vi "Acq-module.vi"(7 "IntermediateFIFO":refnum<k21>="FIFO0", 8 "NumChannels":T1, 9 "SamplingRate0":u16=10000, 11 "Cluster in":T3) -> (3 "cluster out":T4)   [LabVIEW 2013]
uses:
  ctl.ctl
  N Channels.ctl
  <vilib>/rvi/DataTransferAndStorage/Container/Common/niFpgaContainerExecOnDevCompGetState.vi
  <vilib>/rvi/FIFO/Fifo_Resource/nirvififoEmulationWriteFpgaImpl.vi
  <vilib>/rvi/DataTransferAndStorage/Container/Common/niFpgaContainerGetUniqueNameForEmu.vi
  <vilib>/rvi/interface/RandomDataEmulation/nirviRandomDataFPGAFIFO.vi
  <vilib>/rvi/interface/RandomDataEmulation/niFpgaRandomDataHandleErrors.vi
  <vilib>/rvi/eio/common/nirviEmuReportErrorAndStop.vi
  <vilib>/rvi/Emulation/niFpgaSctlEmulationGetInTimedLoop.vi
  <vilib>/rvi/Emulation/niFpgaProcessEmulError.vi
  GlobalReg.vi
  <vilib>/rvi/eio/common/nirviEmuTemplateMethod_errors.vi
  <vilib>/rvi/DataTransferAndStorage/Container/XNode/niFpgaContainer.xnode
  <vilib>/rvi/FIFO/Fifo_Resource/niFpgaFifoEmulationRefIn.vi
  <vilib>/eio/EIONode/EIONode.xnode
panel:
  out "Analog Out Cluster":T2
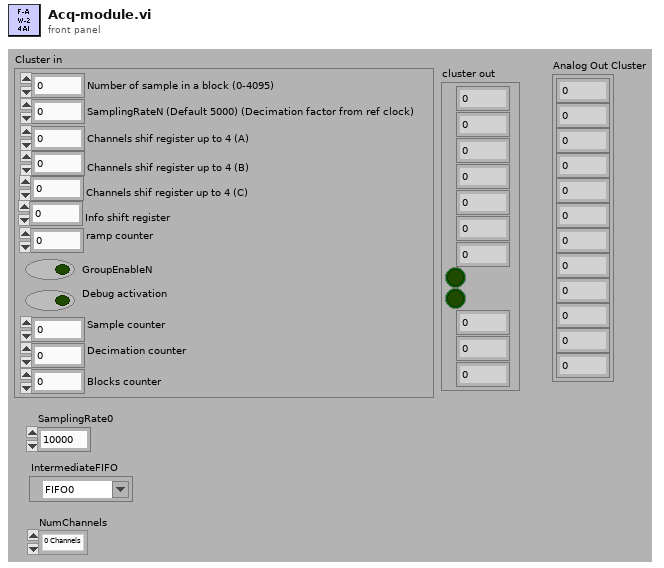
[diagram p1: front panel]
types:
  T1 = typedef "N Channels.ctl" = enum16{"0 Channels", "1 Channels", "2 Channels", "3 Channels", "4 Channels", "5 Channels", "6 Channels", "7 Channels", "8 Channels", "9 Channels", "10 Channels", "11 Channels", "12 Channels"}
  T2 = cluster{i16, i16, i16, i16, i16, i16, i16, i16, i16, i16, i16, i16}
  T3 = typedef "ctl.ctl" = cluster{"Number of sample in a block (0-4095)":u16, "SamplingRateN (Default 5000) (Decimation factor from ref clock)":u16, "Channels shif register up to 4 (A) ":u64, "Channels shif register up to 4 (B) ":u64, "Channels shif register up to 4 (C) ":u64, "Info shift register":u64, "ramp counter":i16, "GroupEnableN":bool, "Debug activation":bool, "Sample counter ":u64, "Decimation counter":u16, "Blocks counter":u16}
  T4 = cluster{u16, u16, u64, u64, u64, u64, i16, bool, bool, u64, u16, u16}
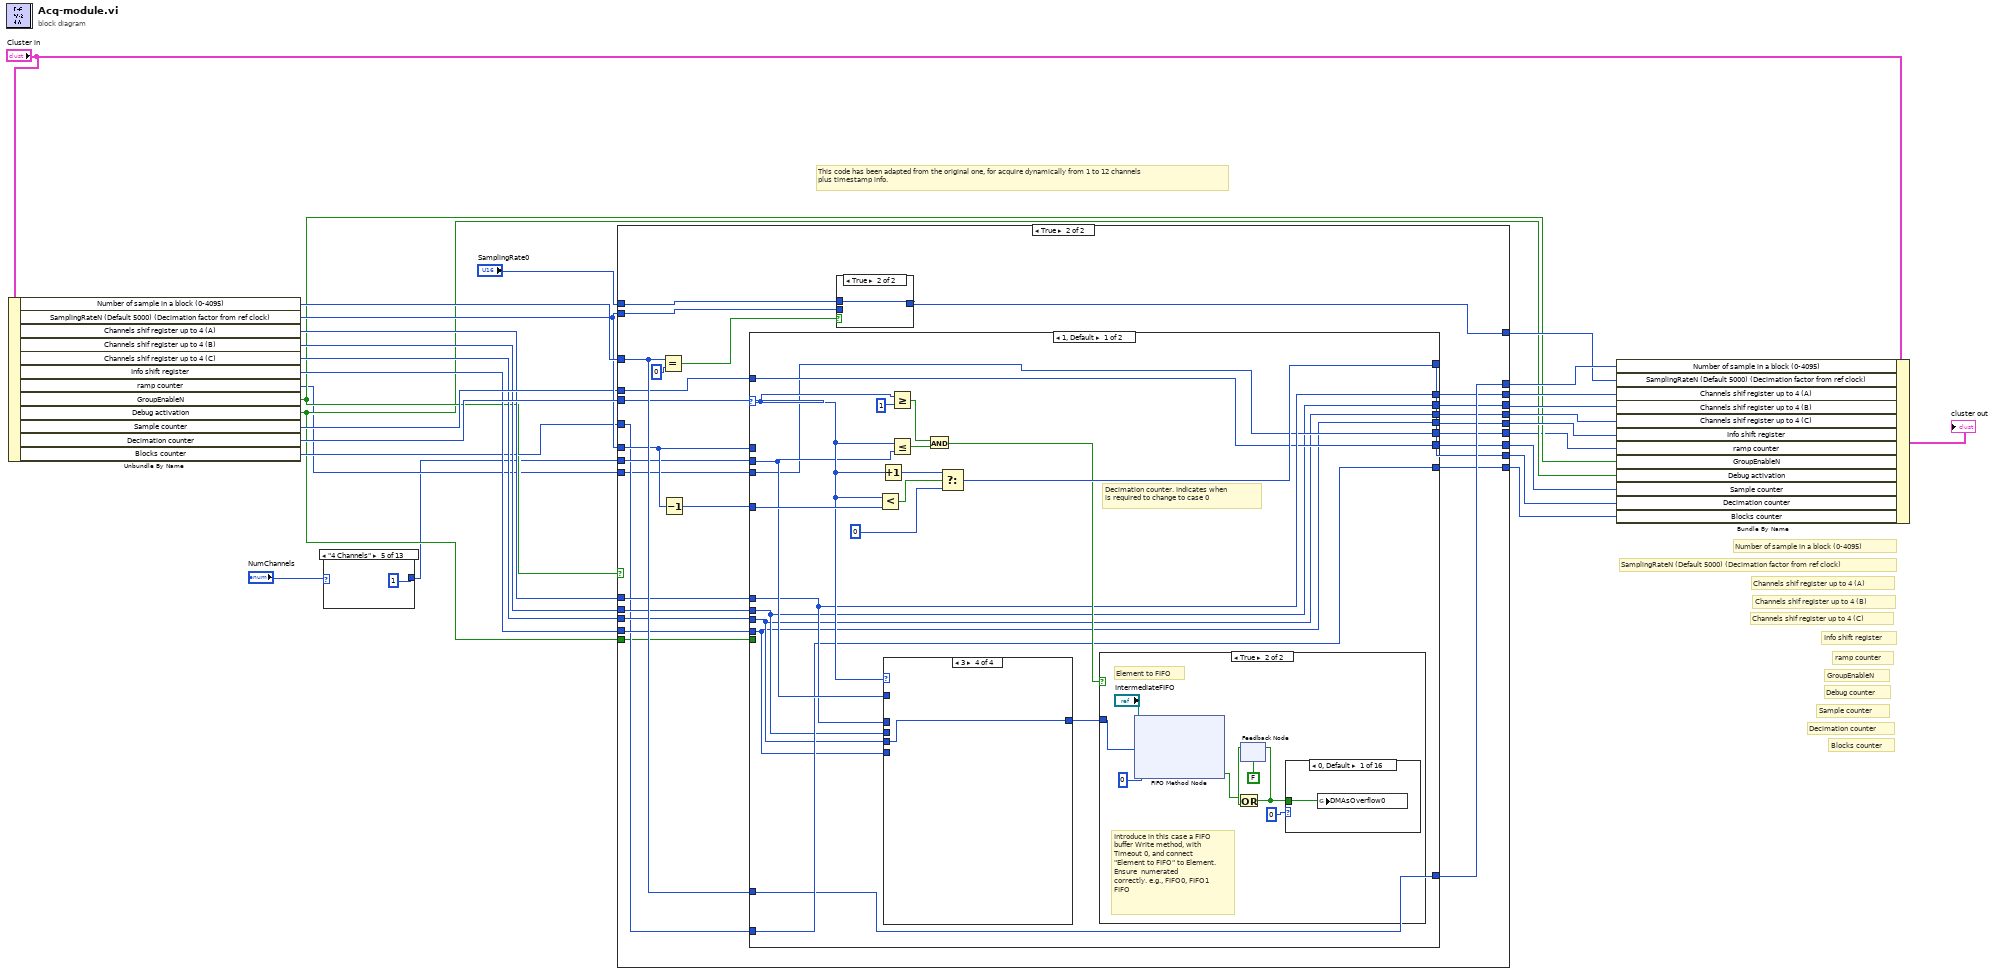
[diagram p0: block diagram]
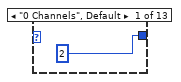
[diagram p2: hidden frame]
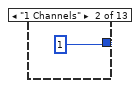
[diagram p3: hidden frame]
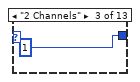
[diagram p4: hidden frame]
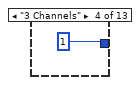
[diagram p5: hidden frame]
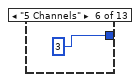
[diagram p6: hidden frame]
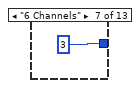
[diagram p7: hidden frame]
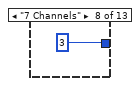
[diagram p8: hidden frame]
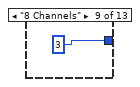
[diagram p9: hidden frame]
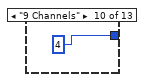
[diagram p10: hidden frame]
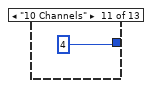
[diagram p11: hidden frame]
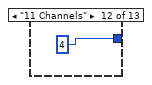
[diagram p12: hidden frame]
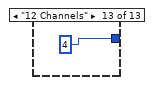
[diagram p13: hidden frame]
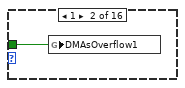
[diagram p16: hidden frame]
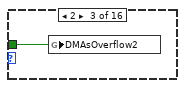
[diagram p17: hidden frame]
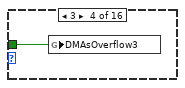
[diagram p18: hidden frame]
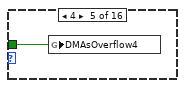
[diagram p19: hidden frame]
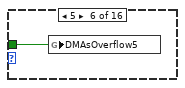
[diagram p20: hidden frame]
diagram:
  # "This code has been adapted from the original one, for acquire dynamically from 1 to 12 channels\nplus timestamp info."
  # "Blocks counter"
  # "Decimation counter"
  # "Sample counter"
  # "Debug counter"
  # "ramp counter"
  # "Info shift register"
  # "Channels shif register up to 4 (C)"
  # "Channels shif register up to 4 (B)"
  # "Channels shif register up to 4 (A)"
  # "SamplingRateN (Default 5000) (Decimation factor from ref clock)"
  # "Number of sample in a block (0-4095)"
  # "GroupEnableN"
  n1 = Unbundle By Name("Cluster in") -> ("Number of sample in a block (0-4095)"=w27:u16, "SamplingRateN (Default 5000) (Decimation factor from ref clock)"=w18:u16, "Channels shif register up to 4 (A)"=w15:u64, "Channels shif register up to 4 (B)"=w14:u64, "Channels shif register up to 4 (C)"=w13:u64, "Info shift register"=w12:u64, "ramp counter"=w7:i16, "GroupEnableN"=w9:bool, "Debug activation"=w8:bool, "Sample counter"=w17:u64, "Decimation counter"=w24:u16, "Blocks counter"=w11:u16)
  n2 = case shown="\"4 Channels\"" "NumChannels" {
    tunnel: [u8 2 ("Number of words") u8 1 ("Number of words") u8 1 ("Number of words") u8 1 ("Number of words") u8 1 ("Number of words") u8 3 ("Number of words") u8 3 ("Number of words") u8 3 ("Number of words") u8 3 ("Number of words") u8 4 ("Number of words") u8 4 ("Number of words") u8 4 ("Number of words") u8 4 ("Number of words")] -> w5
    frame "0 Channels", Default {
    }
    frame "1 Channels" {
    }
    frame "2 Channels" {
    }
    frame "3 Channels" {
    }
    frame "4 Channels" {
    }
    frame "5 Channels" {
    }
    frame "6 Channels" {
    }
    frame "7 Channels" {
    }
    frame "8 Channels" {
    }
    frame "9 Channels" {
    }
    frame "10 Channels" {
    }
    frame "11 Channels" {
    }
    frame "12 Channels" {
    }
  }
  n3 = case shown="True" w9 {
    tunnel: w27 -> [w48 w73]
    tunnel: "SamplingRate0" -> [_ w76]
    tunnel: w18 -> [w49 w74]
    tunnel: [w48 w72] -> w26
    tunnel: [w49 w71] -> w25
    tunnel: w18 -> [_ w70]
    tunnel: w5 -> [_ w68]
    tunnel: w24 -> [w50 w67]
    tunnel: [w50 w66] -> w23
    tunnel: [w47 w65] -> w22
    tunnel: [w46 w64] -> w21
    tunnel: [w45 w63] -> w20
    tunnel: [w44 w62] -> w19
    tunnel: w17 -> [w43 w61]
    tunnel: [w43 w60] -> w16
    tunnel: w15 -> [w47 w59]
    tunnel: w14 -> [w46 w58]
    tunnel: w13 -> [w45 w57]
    tunnel: w12 -> [w44 w56]
    tunnel: w11 -> [w42 w55]
    tunnel: [w42 w54] -> w10
    tunnel: w8 -> [_ w53]
    tunnel: w7 -> [w41 w52]
    tunnel: [w41 w51] -> w6
    frame False {
    }
    frame True {
      n4 = Equal?(x=w73, y=u16 0) -> (x = y?=w75:bool)
      n5 = Decrement(x=w70) -> (x-1=w69:u16)
      n6 = case shown="1, Default" w67 {
        selector: w67 -> [w89 w127]
        tunnel: w73 -> [w82 w158]
        tunnel: [w82 w154] -> w72
        tunnel: w70 -> [_ w151]
        tunnel: w69 -> [w92 _]
        tunnel: w68 -> [w88 _]
        tunnel: [w91 w126] -> w66
        tunnel: [w86 w138] -> w65
        tunnel: [w80 _] -> w64
        tunnel: [w79 _] -> w63
        tunnel: [w78 w137] -> w62
        tunnel: w61 -> [w84 w135]
        tunnel: [w84 w134] -> w60
        tunnel: w59 -> [w86 _]
        tunnel: w58 -> [w80 _]
        tunnel: w57 -> [w79 _]
        tunnel: w56 -> [w78 _]
        tunnel: w55 -> [w83 w133]
        tunnel: [w83 w132] -> w54
        tunnel: w53 -> [_ w131]
        tunnel: w52 -> [w81 w130]
        tunnel: [w81 w129] -> w51
        frame 1, Default {
          # "Decimation counter. Indicates when \nis required to change to case 0"
          n7 = Less?(x=w89, y=w92) -> (x < y?=w85:bool)
          n8 = Increment(x=w89) -> (x+1=w97:u16)
          n9 = case shown="3" w89 {
            tunnel: [u64 0 ("Element") w123 w124 w125] -> w90
            tunnel: w86 -> [_ w123 _ _]
            tunnel: w80 -> [_ _ w124 _]
            tunnel: w79 -> [_ _ _ w125]
            tunnel: w78 -> [_ _ _ _]
            tunnel: w88 -> [_ _ _ _]
            frame Default {
            }
            frame 1 {
            }
            frame 2 {
            }
            frame 3 {
            }
          }
          n10 = Greater Or Equal?(x=w89, y=u16 1) -> (x >= y?=w94:bool)
          n11 = Less Or Equal?(x=w89, y=w88) -> (x <= y?=w93:bool)
          n12 = And(x=w94, y=w93) -> (x .and. y?=w87:bool)
          n13 = Select(t=w97, s=w85, f=u16 0) -> (s? t:f=w91:u16)
          n14 = case shown="True" w87 {
            tunnel: w90 -> [_ w105]
            frame False {
            }
            frame True {
              # "Element to FIFO"
              # "Introduce in this case a FIFO buffer Write method, with Timeout 0, and connect \"Element to FIFO\" to Element. Ensure  numerated\ncorrectly. e.g., FIFO0, FIFO1 \nFIFO"
              n15 = xnode ("FIFO Method Node")("Element"=w105, "Timeout"=0, "FIFO In"="IntermediateFIFO") -> ("Timed Out?"=w98:bool)  [unwired: 1 out]
              n16 = feedback #1(FALSE) -> (w101:bool)
              n17 = Or(x=w98, y=w101) -> (x .or. y?=w100:bool)
              n18 = feedback-in #1(w100) -> ()
              n19 = case shown="0, Default" i16 0 ("DMA number") {
                tunnel: w100 -> [w106 w107 w108 w109 w110 w111 w112 w113 w114 w115 w116 w117 w118 w119 w120 w121]
                frame 0, Default {
                  n20 = global write "GlobalReg.vi" "DMAsOverflow0"(w106) -> ()
                }
                frame 1 {
                  n21 = global write "GlobalReg.vi" "DMAsOverflow1"(w107) -> ()
                }
                frame 2 {
                  n22 = global write "GlobalReg.vi" "DMAsOverflow2"(w108) -> ()
                }
                frame 3 {
                  n23 = global write "GlobalReg.vi" "DMAsOverflow3"(w109) -> ()
                }
                frame 4 {
                  n24 = global write "GlobalReg.vi" "DMAsOverflow4"(w110) -> ()
                }
                frame 5 {
                  n25 = global write "GlobalReg.vi" "DMAsOverflow5"(w111) -> ()
                }
                frame 6 {
                  n26 = global write "GlobalReg.vi" "DMAsOverflow6"(w112) -> ()
                }
                frame 7 {
                  n27 = global write "GlobalReg.vi" "DMAsOverflow7"(w113) -> ()
                }
                frame 8 {
                  n28 = global write "GlobalReg.vi" "DMAsOverflow8"(w114) -> ()
                }
                frame 9 {
                  n29 = global write "GlobalReg.vi" "DMAsOverflow9"(w115) -> ()
                }
                frame 10 {
                  n30 = global write "GlobalReg.vi" "DMAsOverflow10"(w116) -> ()
                }
                frame 11 {
                  n31 = global write "GlobalReg.vi" "DMAsOverflow11"(w117) -> ()
                }
                frame 12 {
                  n32 = global write "GlobalReg.vi" "DMAsOverflow12"(w118) -> ()
                }
                frame 13 {
                  n33 = global write "GlobalReg.vi" "DMAsOverflow13"(w119) -> ()
                }
                frame 14 {
                  n34 = global write "GlobalReg.vi" "DMAsOverflow14"(w120) -> ()
                }
                frame 15 {
                  n35 = global write "GlobalReg.vi" "DMAsOverflow15"(w121) -> ()
                }
              }
            }
          }
        }
        frame 0 {
          n36 = Increment(x=w158) -> (x+1=w155:u16)
          n37 = Less?(x=w155, y=u16 4096) -> (x < y?=w156:bool)
          n38 = To Unsigned Quad Integer(1:w151) -> (0:w153:u64)
          n39 = case shown="True" w156 {
            tunnel: w155 -> [_ w192]
            tunnel: [u16 0 w192] -> w154
            tunnel: w133 -> [w189 w191]
            tunnel: [w188 w191] -> w128
            frame False {
              n40 = Increment(x=w189) -> (x+1=w188:u16)
            }
            frame True {
            }
          }
          n41 = And(x=w153, y=i16 16383) -> (x .and. y?=w150:u64)
          n42 = Logical Shift(y=i8 42, x=w150) -> (x << y=w146:u64)
          n43 = And(x=w135, y=u64 4398046511103) -> (x .and. y?=w147:u64)
          n44 = Increment(x=w135) -> (x+1=w134:u64)
          n45 = And(x=w128, y=u64 255) -> (x .and. y?=w144:u64)
          n46 = Equal?(x=w128, y=u16 255) -> (x = y?=w141:bool)
          n47 = Logical Shift(y=i8 56, x=w144) -> (x << y=w139:u64)
          n48 = Compound Arithmetic op=OR(w147, w146, w139) -> (w136:u64)
          n49 = case shown="False" w131 {
            tunnel: [w160 w180] -> w138
            tunnel: [w159 w187] -> w137
            tunnel: w136 -> [w159 w187]
            tunnel: w130 -> [w162 _]
            tunnel: [w161 i16 0] -> w129
            frame True {
              n50 = Add(x=w162, y=i16 5) -> (x+y=w169:i16)
              n51 = Add(x=i16 10, y=w162) -> (x+y=w167:i16)
              n52 = Add(x=w162, y=i16 15) -> (x+y=w165:i16)
              n53 = Less?(x=w162, y=i16 4095) -> (x < y?=w163:bool)
              n54 = Join Numbers(hi=w162, lo=w169) -> ((hi.lo)=w172:u32)
              n55 = Join Numbers(hi=w167, lo=w165) -> ((hi.lo)=w171:u32)
              n56 = Join Numbers(hi=w172, lo=w171) -> ((hi.lo)=w160:u64)
              n57 = case shown="True" w163 {
                tunnel: w162 -> [_ w175]
                tunnel: [i16 0 w174] -> w161
                frame False {
                }
                frame True {
                  n58 = Increment(x=w175) -> (x+1=w174:i16)
                }
              }
            }
            frame False {
              w184 = i16 427
              # "TODO. For test the AIN\nRegisters"
              # "CH0"
              # "CH1"
              # "CH2"
              # "CH3"
              # "INFO"
              n59 = xnode "I/O Node"() -> ("IO Module\\AI 1 Data N"=w179:i16)  [unwired: 1 in, 1 out]
              n60 = xnode "I/O Node"() -> ("IO Module\\AI 0 Data N"=w178:i16)  [unwired: 1 in, 1 out]
              n61 = global read "GlobalReg.vi" "SimulatedAO0"() -> (w176:i16)
              n62 = global read "GlobalReg.vi" "SimulatedAO1"() -> (w177:i16)
              n63 = Bundle(cluster=T2 {0, 0, 0, 0, 0, 0, 0, 0, 0, 0, 0, 0} ("Cluster 2"), w184, w184, w184, w184, w184, w184, w184, w184, w184, w184, w184, w184) -> (→"Analog Out Cluster":T2)
              n64 = Join Numbers(hi=w177, lo=w176) -> ((hi.lo)=w182:u32)
              n65 = Join Numbers(hi=w179, lo=w178) -> ((hi.lo)=w181:u32)
              n66 = Join Numbers(hi=w182, lo=w181) -> ((hi.lo)=w180:u64)
            }
          }
          n67 = Select(t=u16 0, s=w141, f=w128) -> (s? t:f=w132:u16)
          n68 = Increment(x=w127) -> (x+1=w126:u16)
        }
      }
      n69 = case shown="True" w75 {
        tunnel: w76 -> [_ w194]
        tunnel: [w193 w194] -> w71
        tunnel: w74 -> [w193 _]
        frame False {
        }
        frame True {
        }
      }
    }
  }
  n70 = Bundle By Name(cluster="Cluster in", "Number of sample in a block (0-4095)"=w26, "SamplingRateN (Default 5000) (Decimation factor from ref clock)"=w25, "Channels shif register up to 4 (A)"=w22, "Channels shif register up to 4 (B)"=w21, "Channels shif register up to 4 (C)"=w20, "Info shift register"=w19, "ramp counter"=w6, "GroupEnableN"=w9, "Debug activation"=w8, "Sample counter"=w16, "Decimation counter"=w23, "Blocks counter"=w10) -> (→"cluster out":T3)
